vi "read.vi"(8 "error in (no error)":errorcluster, 11 "IConnection in":refnum<class "IConnection.lvclass">) -> (0 "error out":errorcluster, 2 "message":string, 3 "IConnection out":refnum<class "IConnection.lvclass">)   [LabVIEW 2023, in "IConnection.lvclass"]
uses:
  IConnection.lvclass
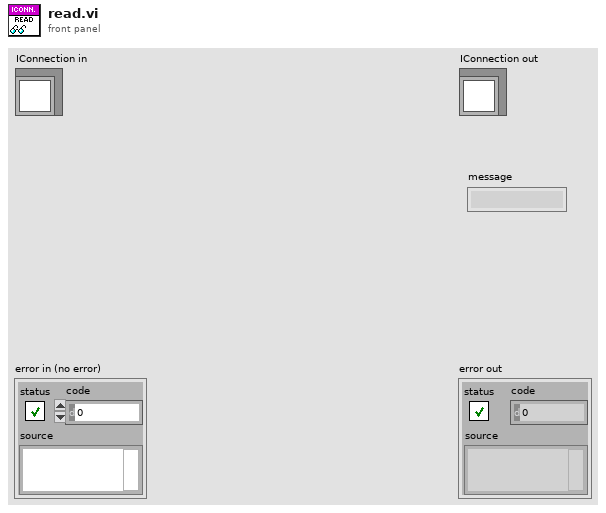
[diagram p1: front panel]
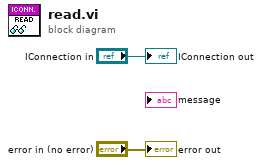
[diagram p0: block diagram]
diagram:
  "error out" <- "error in (no error)"
  "IConnection out" <- "IConnection in"
